vi "HSVColors.vi"() -> ()   [LabVIEW 2021]
panel:
  out "V":picture
  out "S":picture
  out "H":picture
  in  "Path":path
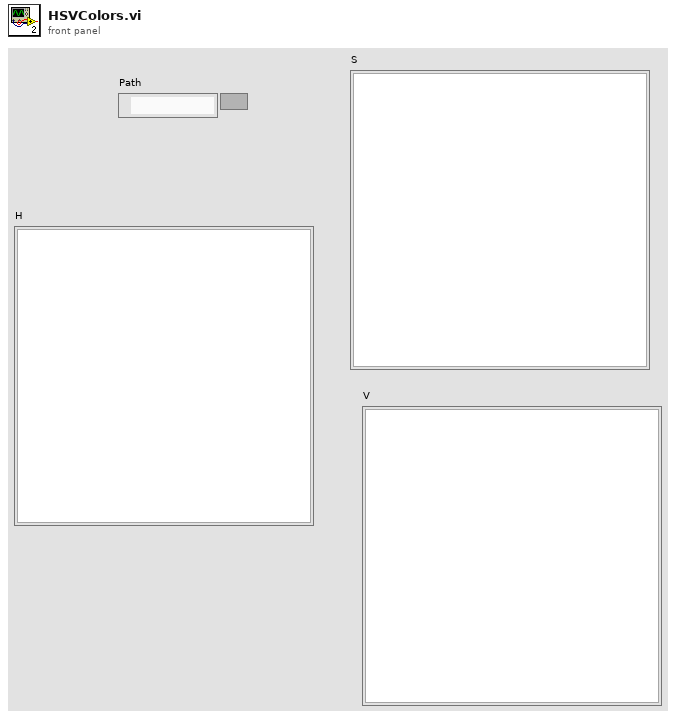
[diagram p1: front panel]
types:
  T1 = typedef "imagedata.ctl" = cluster{"image type":i32, "image depth":i32, "image":u8[], "mask":u8[], "colors":u32[], "Rectangle":cluster{"left":i16, "top":i16, "right":i16, "bottom":i16}}
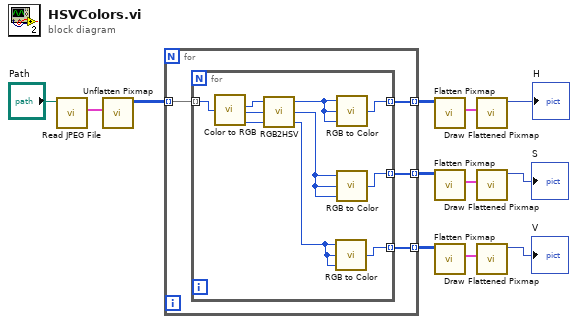
[diagram p0: block diagram]
diagram:
  n1 = call <vilib>:"Read JPEG File.vi"("path to JPEG file"="Path") -> ("image data"=w11:T1)  [unwired: 8 in, 2 out]
  n2 = call <vilib>:"Unflatten Pixmap.vi"("image data"=w11) -> ("24-bit pixmap"=w1:u32[][])  [unwired: 4 in, 6 out]
  n3 = for {
    tunnel: w1 -> [w16] mode=indexing
    tunnel: [w15] -> w8 mode=indexing
    tunnel: [w14] -> w7 mode=indexing
    tunnel: [w13] -> w2 mode=indexing
    n4 = for {
      tunnel: w16 -> [w17] mode=indexing
      tunnel: [w26] -> w15 mode=indexing
      tunnel: [w20] -> w14 mode=indexing
      tunnel: [w18] -> w13 mode=indexing
      n5 = call <vilib>:"Color to RGB.vi"("Color"=w17) -> ("R"=w25:u8, "G"=w24:u8, "B"=w23:u8)  [unwired: 1 out]
      n6 = call <instrlib>:"RGB2HSV.vi"("B"=w23, "G"=w24, "R"=w25) -> ("V"=w19:u8, "S"=w21:u8, "H"=w22:u8)
      n7 = call <vilib>:"RGB to Color.vi"("B"=w19, "G"=w19, "R"=w19) -> ("Color"=w18:u32)
      n8 = call <vilib>:"RGB to Color.vi"("B"=w22, "G"=w22, "R"=w22) -> ("Color"=w26:u32)
      n9 = call <vilib>:"RGB to Color.vi"("B"=w21, "G"=w21, "R"=w21) -> ("Color"=w20:u32)
    }
  }
  n10 = call <vilib>:"Flatten Pixmap.vi"("24-bit pixmap"=w8) -> ("image data"=w10:T1)  [unwired: 10 in]
  n11 = call <vilib>:"Flatten Pixmap.vi"("24-bit pixmap"=w7) -> ("image data"=w5:T1)  [unwired: 10 in]
  n12 = call <vilib>:"Flatten Pixmap.vi"("24-bit pixmap"=w2) -> ("image data"=w3:T1)  [unwired: 10 in]
  n13 = call <vilib>:"Draw Flattened Pixmap.vi"("image data"=w10) -> ("new picture"=→"H":picture)  [unwired: 8 in]
  n14 = call <vilib>:"Draw Flattened Pixmap.vi"("image data"=w5) -> ("new picture"=→"S":picture)  [unwired: 8 in]
  n15 = call <vilib>:"Draw Flattened Pixmap.vi"("image data"=w3) -> ("new picture"=→"V":picture)  [unwired: 8 in]
